vi "APS get feeder running index.vi"(8 "error in (no error)":errorcluster caption="错误输入（无错误）", 10 "Index":i32, 11 "GroupId":i32) -> (0 "error out":errorcluster caption="错误输出", 2 "Index out":i32, 3 "function return":i32)   [LabVIEW 2011, in "APS168.lvlib"]
doc: "I32 FNTYPE APS_get_feeder_running_index( I32 GroupId, I32 *Index );"
uses:
  APS168.lvlib
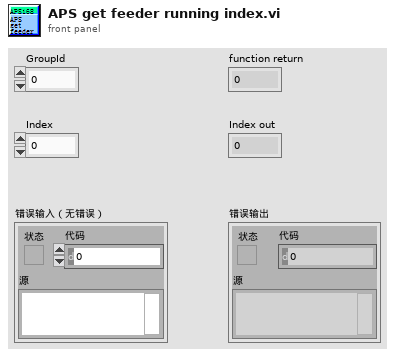
[diagram p1: front panel]
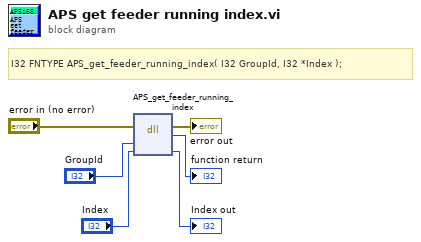
[diagram p0: block diagram]
diagram:
  # "I32 FNTYPE APS_get_feeder_running_index( I32 GroupId, I32 *Index );"
  n1 = dll-call lib="PTH1Labs E软件ADLINK 204CAPS_1_7_1_LIB line 连续运动204APS168.*" fn="APS_get_feeder_running_index"(error in="error in (no error)", "GroupId"="GroupId", "Index"="Index") -> (error out=→"error out":errorcluster, →"function return":i32, "Index"=→"Index out":i32)  [unwired: 3 in, 1 out]
